vi "LJM logger open constants to string.vi"(4 "ConnType":i32, 5 "DevType":i32) -> (1 "ConnTypeString":string, 2 "DevTypeString":string)   [LabVIEW 2026]
panel:
  # "Be sure to change LJM logger open with invalid device filter.vi and LJM logger get error open params.vi if you change this VI."
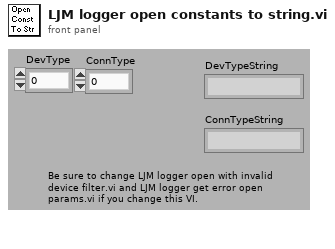
[diagram p1: front panel]
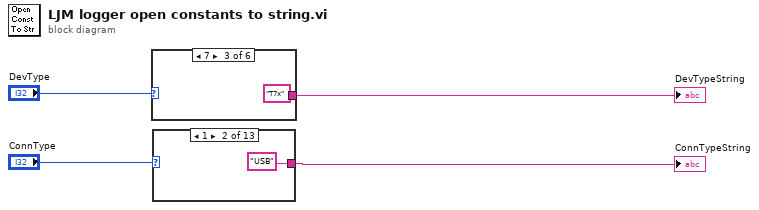
[diagram p0: block diagram]
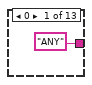
[diagram p2: hidden frame]
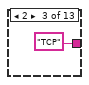
[diagram p3: hidden frame]
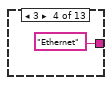
[diagram p4: hidden frame]
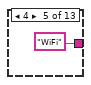
[diagram p5: hidden frame]
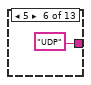
[diagram p6: hidden frame]
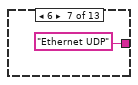
[diagram p7: hidden frame]
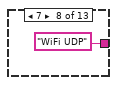
[diagram p8: hidden frame]
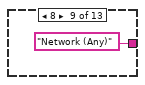
[diagram p9: hidden frame]
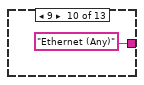
[diagram p10: hidden frame]
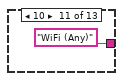
[diagram p11: hidden frame]
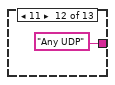
[diagram p12: hidden frame]
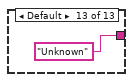
[diagram p13: hidden frame]
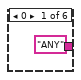
[diagram p14: hidden frame]
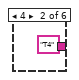
[diagram p15: hidden frame]
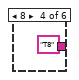
[diagram p16: hidden frame]
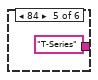
[diagram p17: hidden frame]
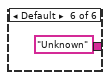
[diagram p18: hidden frame]
diagram:
  n1 = case shown="7" "DevType" {
    tunnel: ["ANY" "T4" "T7x" "T8" "T-Series" "Unknown"] -> w3
    frame 0 {
    }
    frame 4 {
    }
    frame 7 {
    }
    frame 8 {
    }
    frame 84 {
    }
    frame Default {
    }
  }
  "DevTypeString" <- w3
  n2 = case shown="1" "ConnType" {
    tunnel: ["ANY" "USB" "TCP" "Ethernet" "WiFi" "UDP" "Ethernet UDP" "WiFi UDP" "Network (Any)" "Ethernet (Any)" "WiFi (Any)" "Any UDP" "Unknown"] -> w1
    frame 0 {
    }
    frame 1 {
    }
    frame 2 {
    }
    frame 3 {
    }
    frame 4 {
    }
    frame 5 {
    }
    frame 6 {
    }
    frame 7 {
    }
    frame 8 {
    }
    frame 9 {
    }
    frame 10 {
    }
    frame 11 {
    }
    frame Default {
    }
  }
  "ConnTypeString" <- w1
